vi "Configure Reference Levels.vi"(5 "Low Reference (10.0%)":dbl=10.0, 7 "Mid Reference (50.0%)":dbl=50.0, 8 "error in (no error)":errorcluster, 9 "High Reference (90.0%)":dbl=90.0, 10 "Channel (15: All Waveforms)":i32(ring)=15 items=["Channel 1"=1, "Channel 2"=2, "Channel 3"=3, "Channel 4"=4, "Function 1"=5, "Function 2"=6, "Function 3"=7, "Function 4"=8, "Memory 1"=9, "Memory 2"=10, "Memory 3"=11, "Memory 4"=12, "All Waveforms"=15], 11 "VISA resource name":refnum<visa-resource-name>) -> (0 "error out":errorcluster, 3 "VISA resource name out":refnum<visa-resource-name>)   [LabVIEW 2020, in "Agilent 90000 Series.lvlib"]
doc: "Configures the reference levels in percents for waveform measurements. \n\nYou must call this VI before you call the Read Waveform Measurement VI or Fetch Waveform Measurement VI to take a rise time, fall time, width negative, width positive, duty cycle negative, or duty cycle positive measurement."
uses:
  Agilent 90000 Series.lvlib
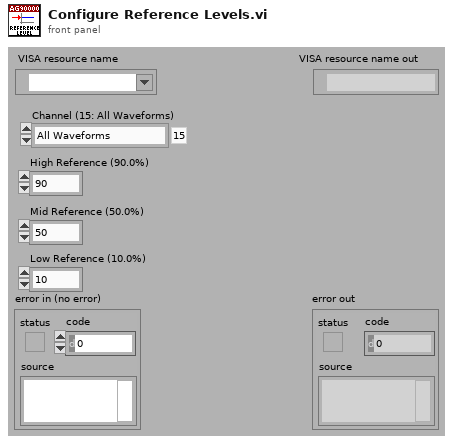
[diagram p1: front panel]
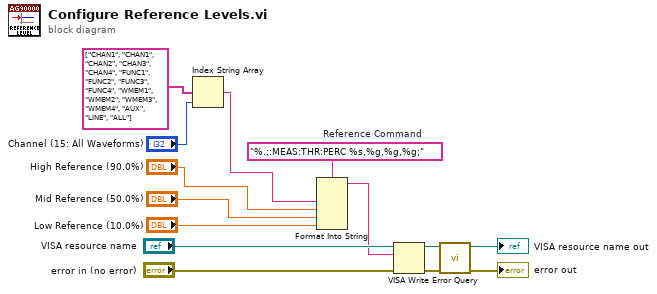
[diagram p0: block diagram]
diagram:
  w8 = "%.;:MEAS:THR:PERC %s,%g,%g,%g;"  # Reference Command
  n1 = Index String Array(1:"Channel (15: All Waveforms)", 2:string[] ["CHAN1", "CHAN1", "CHAN2", "CHAN3", "CHAN4", "FUNC1", "FUNC2", "FUNC3", "FUNC4", "WMEM1", "WMEM2", "WMEM3", "WMEM4", "AUX", "LINE", "ALL"] ("subarray 2")) -> (0:w5:string)  [unwired: 1 out]
  n2 = Format Into String(format string=w8, w5, "High Reference (90.0%)", "Mid Reference (50.0%)", "Low Reference (10.0%)") -> (resulting string=w7:string)  [unwired: 2 in, 1 out]
  n3 = VISA Write(VISA resource name="VISA resource name", write buffer=w7, error in (no error)="error in (no error)") -> (VISA resource name out=w10:refnum<visa-resource-name>, error out=w9:errorcluster)  [unwired: 1 out]
  n4 = call "Error Query.vi"("error in (no error)"=w9, "VISA resource name"=w10) -> ("error out"=→"error out":errorcluster, "VISA resource name out"=→"VISA resource name out":refnum<visa-resource-name>)  [unwired: 8 out]
